vi "二维数组非空行数.vi"(1 "数组":string[][](array[string])) -> (0 "行数":i32)   [LabVIEW 2015]
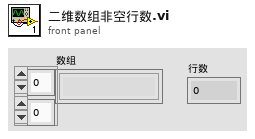
[diagram p1: front panel]
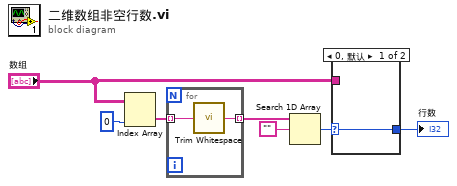
[diagram p0: block diagram]
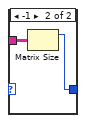
[diagram p2: hidden frame]
diagram:
  n1 = Index Array(array="数组", index (col)=0 ("禁用的索引 (列)")) -> (element=w6:string[])  [unwired: 1 in]
  n2 = for {
    tunnel: w6 -> [w9] mode=indexing
    tunnel: [w8] -> w4 mode=indexing
    n3 = call <vilib>:"Trim Whitespace.vi"("string"=w9) -> ("trimmed string"=w8:string)  [unwired: 1 in]
  }
  n4 = Search 1D Array(1D array=w4, element="") -> (index of element=w3:i32)  [unwired: 1 in]
  n5 = case shown="0, 默认" w3 {
    selector: w3 -> [w10 _]
    tunnel: "数组" -> [_ w12]
    tunnel: [w10 w11] -> w2
    frame 0, Default {
    }
    frame -1 {
      n6 = Matrix Size(0:w12) -> (1:w11:i32)  [unwired: 1 out]
    }
  }
  "行数" <- w2
